vi "Table, Copy Column Widths.vi"(4 "error in":errorcluster, 6 "Tbl Refnum Dst":refnum<vi>, 7 "Tbl Refnum Src":refnum<vi>) -> (0 "error out":errorcluster, 2 "Tbl Refnum Dst out":refnum<vi>, 3 "Tbl Refnum Src out":refnum<vi>)   [LabVIEW 2010]
doc: "Copies the column width attributes of the source table to the destination table."
uses:
  <vilib>/Utility/miscctls.llb/LVRowAndColumnTypeDef.ctl
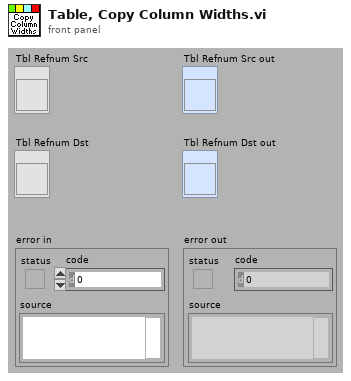
[diagram p1: front panel]
types:
  T1 = typedef "LVRowAndColumnTypeDef.ctl" = cluster{"Row":i32, "Column":i32}
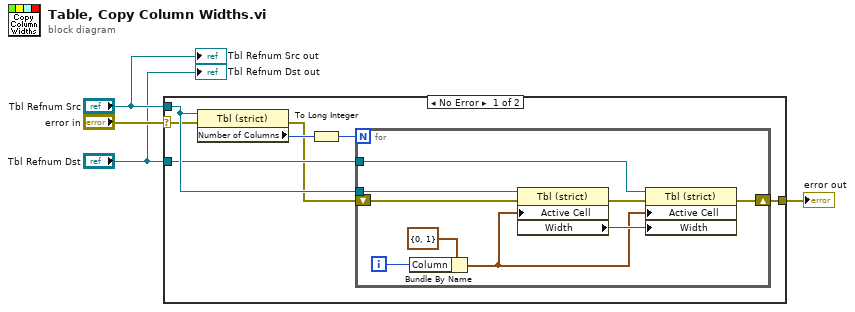
[diagram p0: block diagram]
diagram:
  n1 = case shown="No Error" "error in" {
    selector: "error in" -> [w5 w21]
    tunnel: "Tbl Refnum Src" -> [w9 _]
    tunnel: "Tbl Refnum Dst" -> [w8 _]
    tunnel: [w6 w21] -> w4
    frame No Error {
      n2 = property class="Tbl (strict)"(reference=w9, error in=w5) -> (error out=w7:errorcluster, "Number of Columns"=w11:u32)  [unwired: 1 out]
      n3 = To Long Integer(number=w11) -> (32bit integer=w10:i32)
      n4 = for {
        N: w10 -> [_]
        tunnel: w9 -> [w20]
        tunnel: w8 -> [w16]
        shift-right: [w13] -> w6
        shift-left: w7 -> [w14]
        i -> [w18]
        n5 = Bundle By Name(cluster=T1 {"Row"=0, "Column"=1} ("Selection Start 2"), "Column"=w18) -> (w15:T1)
        n6 = property class="Tbl (strict)"(reference=w20, error in=w14, "Active Cell"=w15) -> (error out=w12:errorcluster, "Width"=w17:u32)  [unwired: 1 out]
        n7 = property class="Tbl (strict)"(reference=w16, error in=w12, "Active Cell"=w15, "Width"=w17) -> (error out=w13:errorcluster)  [unwired: 1 out]
      }
    }
    frame Error {
    }
  }
  "error out" <- w4
  "Tbl Refnum Src out" <- "Tbl Refnum Src"
  "Tbl Refnum Dst out" <- "Tbl Refnum Dst"
